vi "Decrypt dSpace.vi"(11 "Numeric in":u32) -> (0 "Reset succesful":bool, 1 "Lenkstatus":bool, 2 "wurde eingegriffen?":bool, 3 "Numeric out":u32)   [LabVIEW 2016]
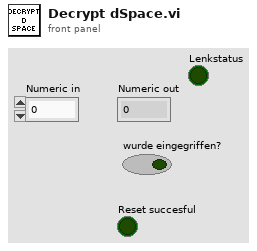
[diagram p1: front panel]
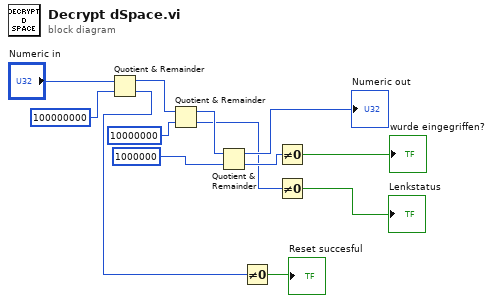
[diagram p0: block diagram]
diagram:
  n1 = Quotient & Remainder(x="Numeric in", y=u32 100000000) -> (x-y*floor(x/y)=w3:u32, floor(x/y)=w2:u32)
  n2 = Quotient & Remainder(x=w3, y=u32 10000000) -> (x-y*floor(x/y)=w8:u32, floor(x/y)=w7:u32)
  n3 = Quotient & Remainder(x=w8, y=u32 1000000) -> (x-y*floor(x/y)=→"Numeric out":u32, floor(x/y)=w10:u32)
  n4 = Not Equal To 0?(x=w2) -> (x != 0?=→"Reset succesful":bool)
  n5 = Not Equal To 0?(x=w10) -> (x != 0?=→"wurde eingegriffen?":bool)
  n6 = Not Equal To 0?(x=w7) -> (x != 0?=→"Lenkstatus":bool)
